vi "Monitor and Configure Time References.vi"() -> ()   [LabVIEW 2019]
doc: "Demonstrates how to monitor and configure IEEE 1588-2008 and IEEE 802.1AS-2011 time references running on a real-time system."
uses:
  <instrlib>/niSync/niSync.llb/niSync Initialize (Default).vi
panel:
  out "Timing:Offset from Time Reference (ns)":dbl
  in  "BMCA Mode":i32(ring) items=["SlaveOnly", "MasterSlave"]
  in  "NI-Sync Resource":tag
  out "Error Out":errorcluster
  in  "stop":bool
  in  "802.1AS:Clock Accuracy":i32(ring)=32 items=["Within25nsec"=32, "Within100nsec"=33, "Within250nsec"=34, "Within1usec"=35, "Within2500nsec"=36, "Within10usec"=37, "Within25usec"=38, "Within100usec"=39, "Within250usec"=40, "Within1msec"=41, "Within2500usec"=42, "Within10msec"=43, "Within25msec"=44, "Within100msec"=45, "Within250msec"=46, "Within1sec"=47, "Within10sec"=48, "GreaterThan10sec"=49, "Unknown"=254]
  in  "Port State":i32(ring)=3 items=["Disabled"=3, "Master"=6, "Passive"=7, "Slave"=9]
  in  "1588:Clock Accuracy":i32(ring) items=["Unknown", "Within25nsec", "Within100nsec", "Within250nsec", "Within1usec", "Within2500nsec", "Within10usec", "Within25usec", "Within100usec", "Within250usec", "Within1msec", "Within2500usec", "Within10msec", "Within25msec", "Within100msec", "Within250msec", "Within1sec", "Within10sec", "GreaterThan10sec"]
  in  "Clock State":i32(ring) items=["Initializing", "Faulty", "Disabled", "Listening", "PreMaster", "Master", "Passive", "Uncalibrated", "Slave", "Stopped"]
  in  "Protocol Tab":T1(tab) caption="System Properties"
  in  "Persist?":bool
  out "802.1AS Monitor":string[][](table)
  in  "802.1AS Time Reference to Configure":i32(ring)
  in  "Priority1":i32=246
  in  "Priority2":i32=247
  in  "Apply 802.1as":bool caption="stop"
  out "802.1AS TAB Monitor":string[][](table)
  in  "Apply 802.1as TAB":bool caption="stop"
  in  "Persist?":bool
  in  "Priority2":i32=247
  in  "Priority1":i32=246
  in  "802.1AS TAB Time Reference to Configure":i32(ring)
  in  "Persist?":bool
  in  "1588 Time Reference to Configure":i32(ring) items=["IEEE 1588-2008_2"]
  in  "Appy 1588":bool caption="stop"
  out "1588 Monitor":string[][](table)
  in  "Priority1":i32=128
  in  "Priority2":i32=128
  in  "BMCA Mode":i32(ring)=1 items=["SlaveOnly", "MasterSlave"]
  out "1588 BC Monitor":string[][](table)
  in  "Appy 1588 BC":bool caption="stop"
  in  "Persist?":bool
  in  "Priority2":i32=128
  in  "Priority1":i32=128
  in  "1588 BC Time Reference to Configure":i32(ring)
  # "Setup"
  # "Overview: Demonstrates how to monitor and configure IEEE 1588-2008 (BC) and IEEE 802.1AS-2011 (TAB)\ntime references running on a real-time system.\nRequirements: Runs on Windows and Linux RT hosts to configure and monitor Linux RT devices.\nInstructions:\n1. Select the resource to monitor/configure in the NI-Sync Resource dropdown.\n2. Select the desired polling interval for monitoring.\n3. Use the tabs to switch to the protcol of interest.\n4. Monitor the enabled time references of this type in the table.\n5. To configure properties of a time reference:\n     a) Select the 1588 Time Reference to Configure.\n     b) Set properties to desired values.\n     c) Enable the Persist? Boolean if you would like these settings to persist across reboots.\n     d) Select Apply to commit the desired settings."
  # "IEEE 802.1AS-2011 is a network-based time synchronization protocol that is similar to IEEE 1588-2008, but is optimized for time-sensitive applications. It also provides fewer configuration options and\nrequires 802.1AS-compatible network infrastructure. Each instance of IEEE 802.1AS-2011 is associated with a single network interface on the real-time system, and each can be either a slave to the\nnetwork's grandmaster or the grandmaster to a network of devices."
  # "IEEE 802.1AS-2011 TAB (time-aware bridge) is like IEEE 802.1AS-2011, except each instance of IEEE 802.1AS-2011 TAB is associated with multiple ports, typically on a device that acts as a network switch."
  # "IEEE 1588-2008 is a network-based time synchronization protocol (also refered to as PTP) that synchronized devices to a single grandmaster clock. Each instance of IEEE 1588-2008 is associated with a\nsingle network interface on the real-time system, and each can be either a slave to the network's grandmaster or the grandmaster to a network of devices."
  # "IEEE 1588-2008 BC (boundary clock) is like IEEE 1588-2008, except each instance of IEEE 1588-2008 BC is associated with multiple ports, typically on a device that acts as a network switch."
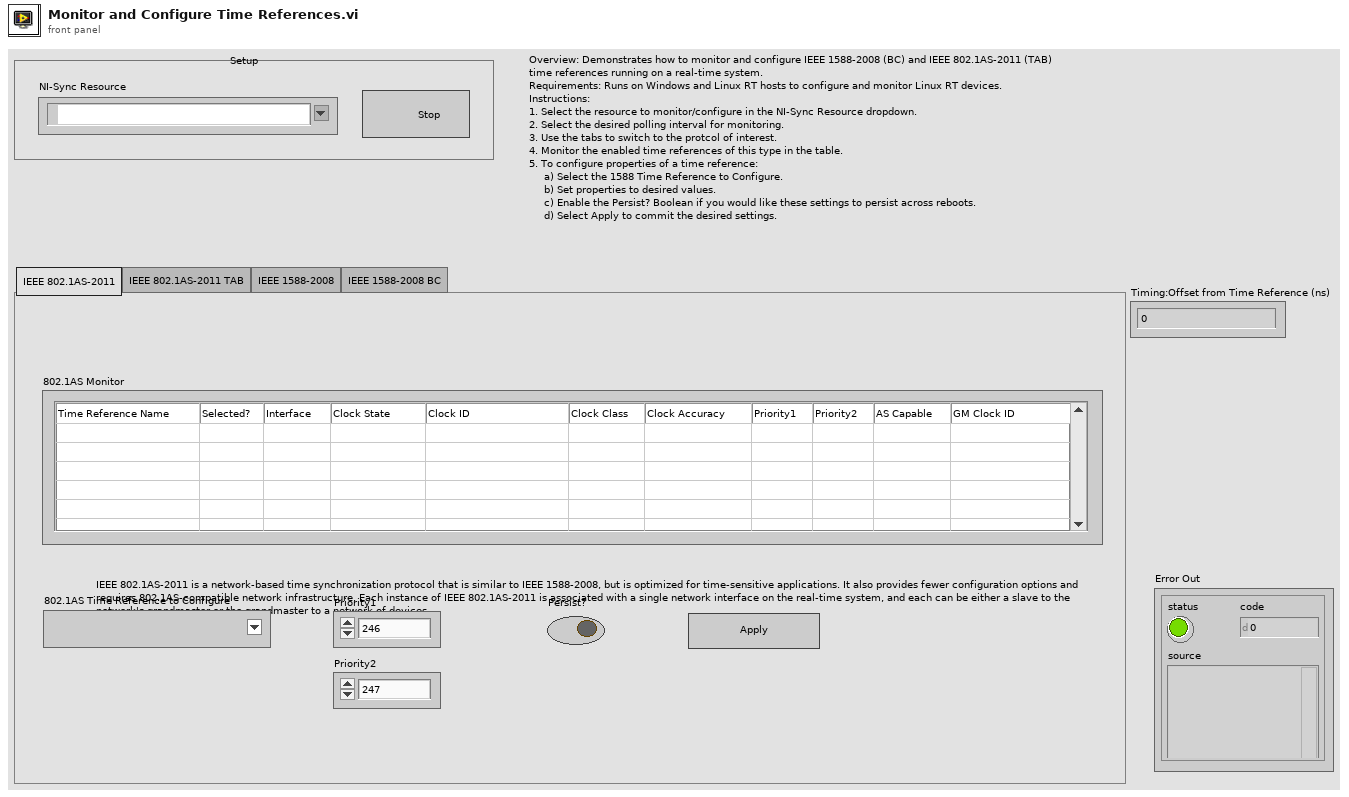
[diagram p1: front panel]
types:
  T1 = enum32{"IEEE 802.1AS-2011", "IEEE 802.1AS-2011 TAB", "IEEE 1588-2008", "IEEE 1588-2008 BC"}
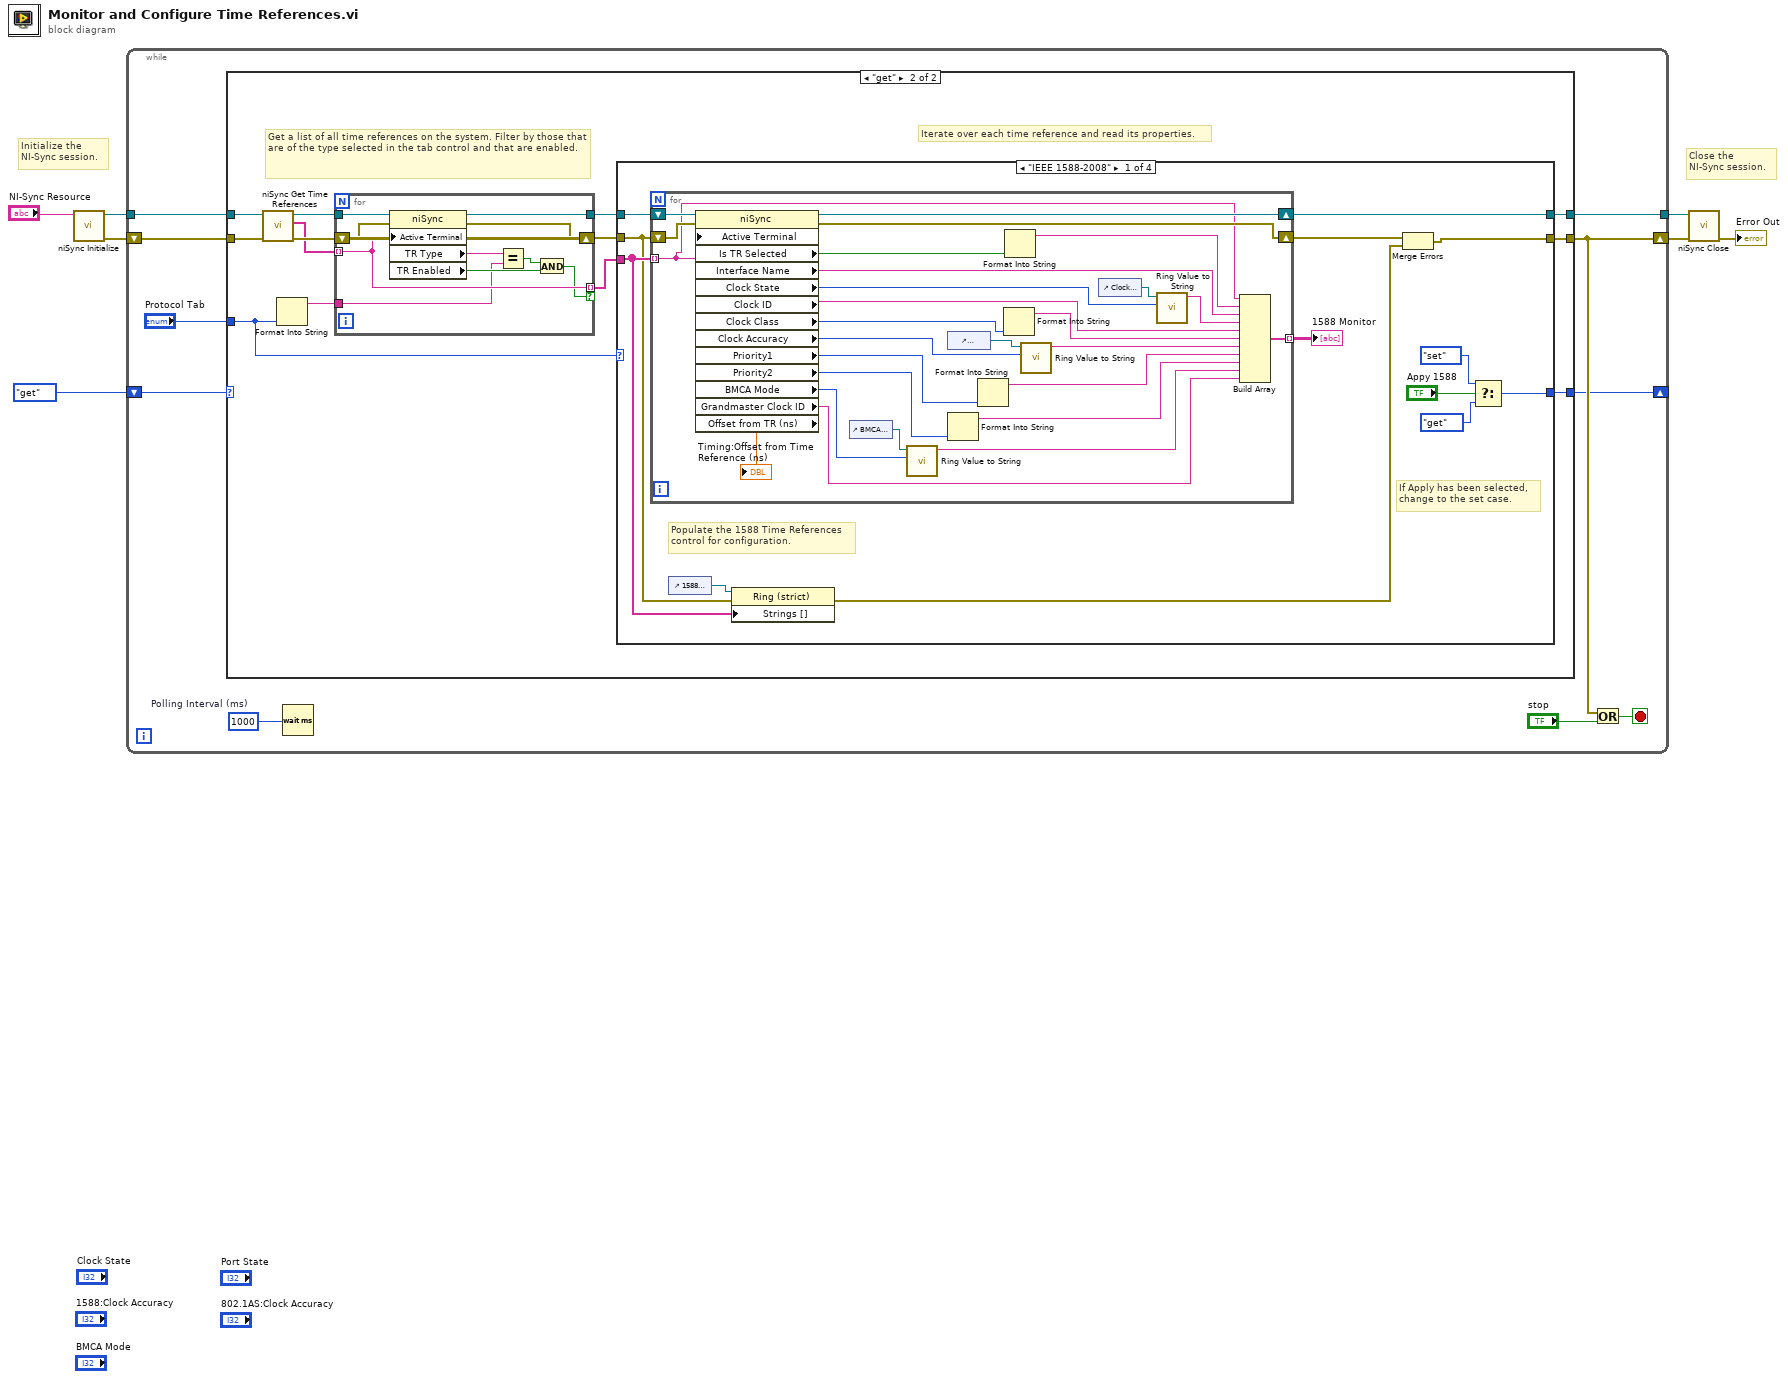
[diagram p0: block diagram]
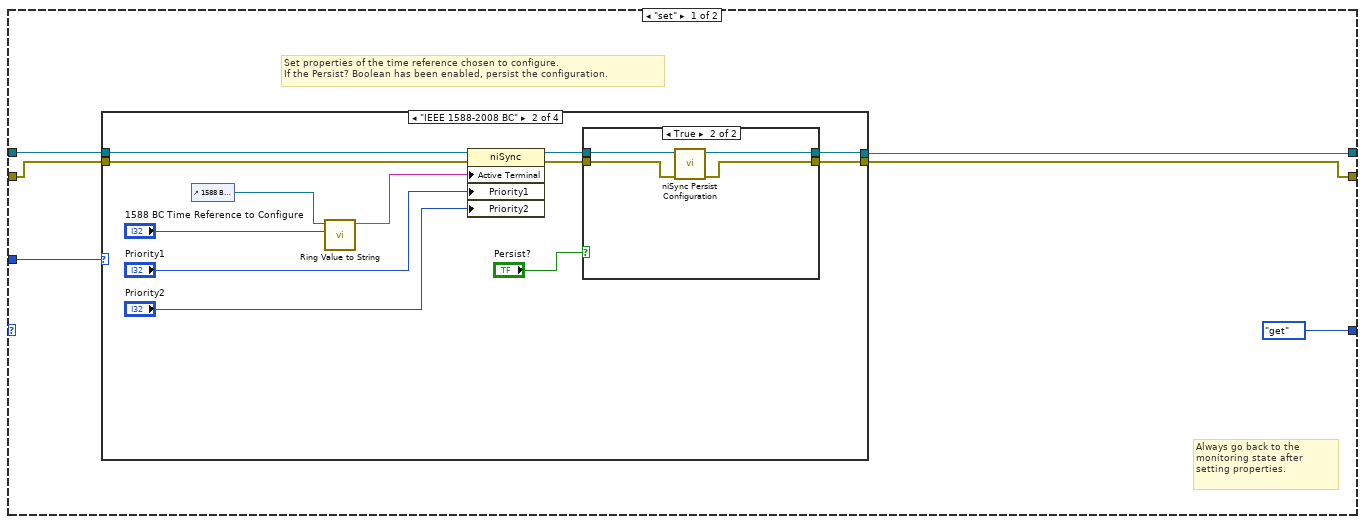
[diagram p2: hidden frame]
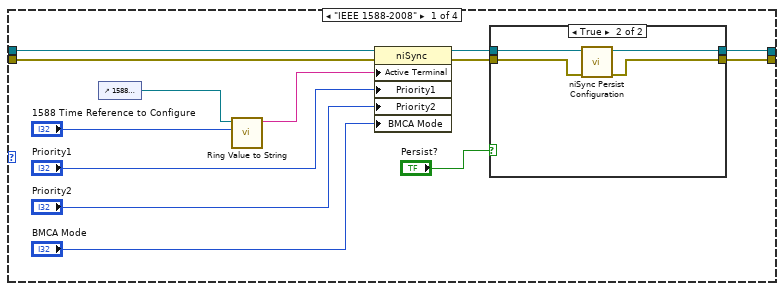
[diagram p3: hidden frame]
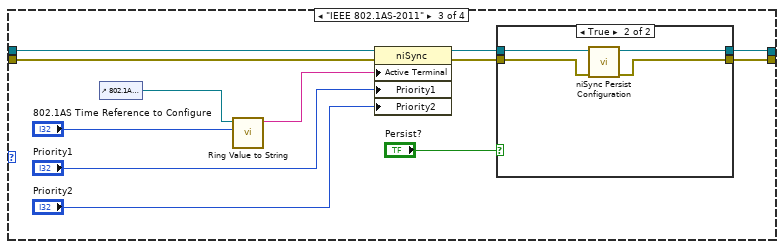
[diagram p6: hidden frame]
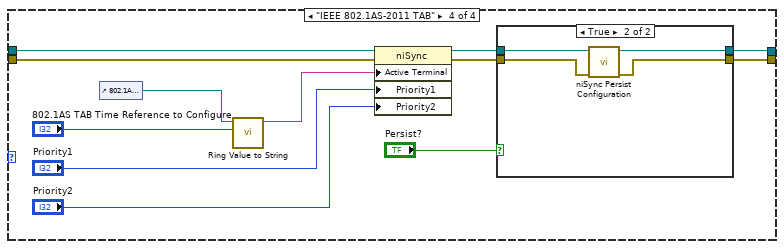
[diagram p8: hidden frame]
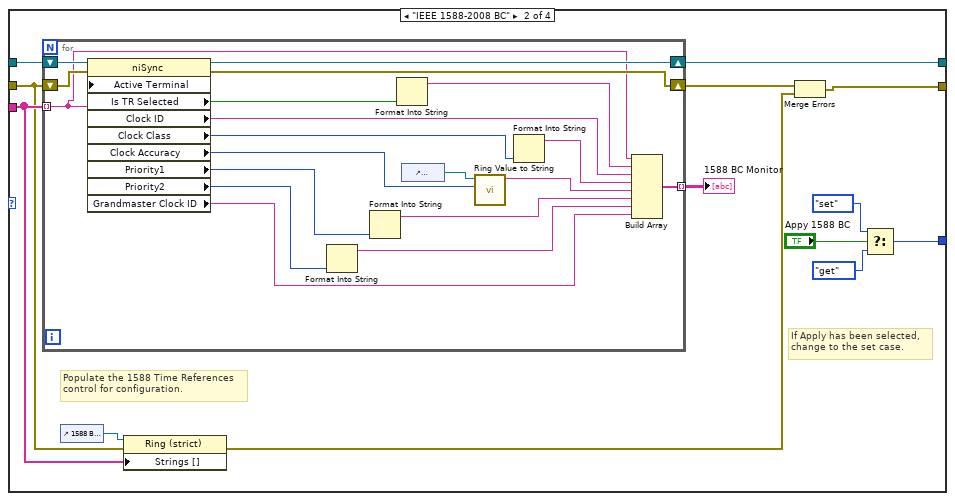
[diagram p10: hidden frame]
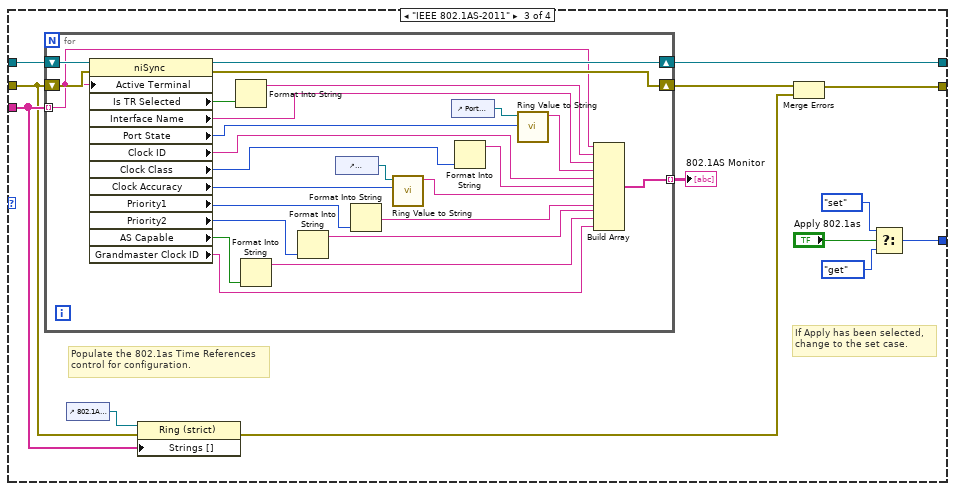
[diagram p11: hidden frame]
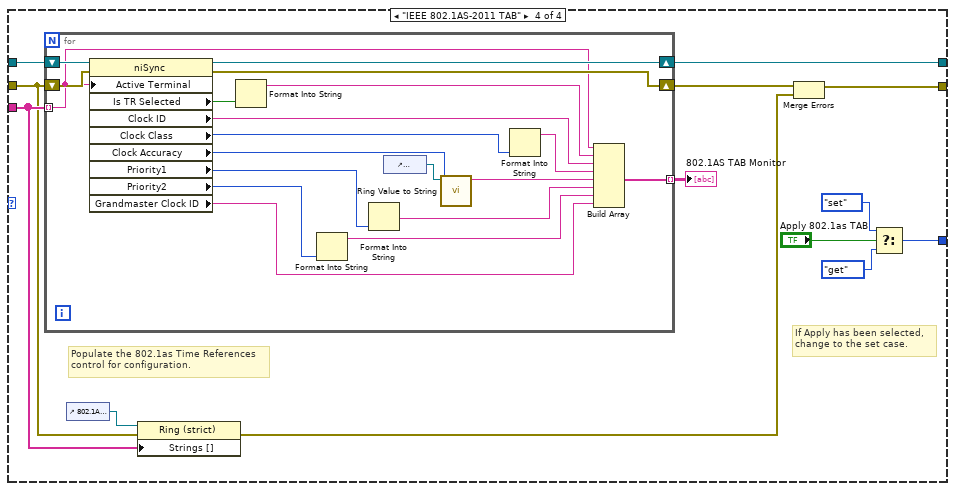
[diagram p12: hidden frame]
diagram:
  # "Close the\nNI-Sync session."
  # "Initialize the\nNI-Sync session."
  n1 = call-poly <instrlib>:"niSync Initialize.vi"("resource name"="NI-Sync Resource") -> ("error out"=w5:errorcluster, "instrument handle out"=w7:refnum<k15>)  [unwired: 9 in]
  n2 = while {
    tunnel: w7 -> [w17]
    tunnel: [w15] -> w6
    shift-right: [w13] -> w4
    shift-left: w5 -> [w16]
    shift-right: [w8] -> _
    shift-left: enum16{"get", "set"}."get" -> [w10]
    stop <- w14 stop-if-true
    w12 = u32 1000  # Polling Interval (ms)
    n3 = case shown="\"get\"" w10 {
      tunnel: w17 -> [w23 w109]
      tunnel: w16 -> [w19 w108]
      tunnel: [w22 w103] -> w15
      tunnel: [w21 w98] -> w13
      tunnel: "Protocol Tab" -> [w20 w99]
      tunnel: [enum16{"get", "set"}."get" w97] -> w8
      frame "set" {
        # "Always go back to the\nmonitoring state after setting properties."
        # "Set properties of the time reference chosen to configure.\nIf the Persist? Boolean has been enabled, persist the configuration."
        n4 = case shown="\"IEEE 1588-2008 BC\"" w20 {
          tunnel: w23 -> [w34 w52 w67 w85]
          tunnel: [w28 w46 w62 w80] -> w22
          tunnel: w19 -> [w30 w48 w66 w84]
          tunnel: [w27 w45 w61 w79] -> w21
          frame "IEEE 1588-2008" {
            n5 = control-ref of="1588 Time Reference to Configure"() -> (w36:refnum<vi>)
            n6 = call "Ring Value to String.vi"("Value"="1588 Time Reference to Configure", "Ring in"=w36) -> ("String"=w33:string)  [unwired: 9 in]
            n7 = property class="niSync"(reference=w34, error in=w30, "Active Terminal"=w33, "Priority1"="Priority1", "Priority2"="Priority2", "BMCA Mode"="BMCA Mode") -> (reference out=w29:refnum<k15>, error out=w26:errorcluster)
            n8 = case shown="True" "Persist?" {
              tunnel: [w38 w42] -> w28
              tunnel: [w37 w41] -> w27
              tunnel: w29 -> [w38 w40]
              tunnel: w26 -> [w37 w39]
              frame False {
              }
              frame True {
                n9 = call <instrlib>:"niSync Persist Configuration.vi"("error in (no error)"=w39, "instrument handle"=w40) -> ("error out"=w41:errorcluster, "instrument handle out"=w42:refnum<k15>)  [unwired: 8 in]
              }
            }
          }
          frame "IEEE 1588-2008 BC" {
            n10 = control-ref of="1588 BC Time Reference to Configure"() -> (w54:refnum<vi>)
            n11 = call "Ring Value to String.vi"("Value"="1588 BC Time Reference to Configure", "Ring in"=w54) -> ("String"=w51:string)  [unwired: 9 in]
            n12 = property class="niSync"(reference=w52, error in=w48, "Active Terminal"=w51, "Priority1"="Priority1", "Priority2"="Priority2") -> (reference out=w47:refnum<k15>, error out=w44:errorcluster)
            n13 = case shown="True" "Persist?" {
              tunnel: [w56 w60] -> w46
              tunnel: [w55 w59] -> w45
              tunnel: w47 -> [w56 w58]
              tunnel: w44 -> [w55 w57]
              frame False {
              }
              frame True {
                n14 = call <instrlib>:"niSync Persist Configuration.vi"("error in (no error)"=w57, "instrument handle"=w58) -> ("error out"=w59:errorcluster, "instrument handle out"=w60:refnum<k15>)  [unwired: 8 in]
              }
            }
          }
          frame "IEEE 802.1AS-2011" {
            n15 = control-ref of="802.1AS Time Reference to Configure"() -> (w72:refnum<vi>)
            n16 = call "Ring Value to String.vi"("Value"="802.1AS Time Reference to Configure", "Ring in"=w72) -> ("String"=w68:string)  [unwired: 9 in]
            n17 = property class="niSync"(reference=w67, error in=w66, "Active Terminal"=w68, "Priority1"="Priority1", "Priority2"="Priority2") -> (reference out=w64:refnum<k15>, error out=w63:errorcluster)
            n18 = case shown="True" "Persist?" {
              tunnel: w64 -> [w74 w78]
              tunnel: w63 -> [w73 w77]
              tunnel: [w74 w76] -> w62
              tunnel: [w73 w75] -> w61
              frame False {
              }
              frame True {
                n19 = call <instrlib>:"niSync Persist Configuration.vi"("error in (no error)"=w77, "instrument handle"=w78) -> ("error out"=w75:errorcluster, "instrument handle out"=w76:refnum<k15>)  [unwired: 8 in]
              }
            }
          }
          frame "IEEE 802.1AS-2011 TAB" {
            n20 = control-ref of="802.1AS TAB Time Reference to Configure"() -> (w90:refnum<vi>)
            n21 = call "Ring Value to String.vi"("Value"="802.1AS TAB Time Reference to Configure", "Ring in"=w90) -> ("String"=w86:string)  [unwired: 9 in]
            n22 = property class="niSync"(reference=w85, error in=w84, "Active Terminal"=w86, "Priority1"="Priority1", "Priority2"="Priority2") -> (reference out=w82:refnum<k15>, error out=w81:errorcluster)
            n23 = case shown="True" "Persist?" {
              tunnel: w82 -> [w92 w96]
              tunnel: w81 -> [w91 w95]
              tunnel: [w92 w94] -> w80
              tunnel: [w91 w93] -> w79
              frame False {
              }
              frame True {
                n24 = call <instrlib>:"niSync Persist Configuration.vi"("error in (no error)"=w95, "instrument handle"=w96) -> ("error out"=w93:errorcluster, "instrument handle out"=w94:refnum<k15>)  [unwired: 8 in]
              }
            }
          }
        }
      }
      frame "get" {
        # "Iterate over each time reference and read its properties."
        # "Get a list of all time references on the system. Filter by those that are of the type selected in the tab control and that are enabled."
        n25 = call <instrlib>:"niSync Get Time References.vi"("error in (no error)"=w108, "instrument handle"=w109) -> ("error out"=w106:errorcluster, "time references"=w105:string[], "instrument handle out"=w107:refnum<k15>)  [unwired: 7 in]
        n26 = Format Into String(w99) -> (resulting string=w100:string)  [unwired: 3 in, 1 out]
        n27 = for {
          tunnel: w107 -> [w261]
          tunnel: w105 -> [w258] mode=indexing
          tunnel: w100 -> [w252]
          tunnel: [w258] -> w104 mode=indexing if=w254
          tunnel: [w257] -> w102
          shift-right: [w253] -> w101
          shift-left: w106 -> [w260]
          n28 = property class="niSync"(reference=w261, error in=w260, "Active Terminal"=w258) -> (reference out=w257:refnum<k15>, error out=w253:errorcluster, "TR Type"=w259:string, "TR Enabled"=w255:bool)
          n29 = Equal?(x=w259, y=w252) -> (x = y?=w256:bool)
          n30 = And(x=w256, y=w255) -> (x .and. y?=w254:bool)
        }
        n31 = case shown="\"IEEE 1588-2008\"" w99 {
          tunnel: w104 -> [w118 w158 w191 w229]
          tunnel: w102 -> [w122 w162 w194 w232]
          tunnel: [w121 w161 w193 w231] -> w103
          tunnel: w101 -> [w115 w155 w186 w224]
          tunnel: [w114 w154 w189 w227] -> w98
          tunnel: [w110 w150 w183 w221] -> w97
          frame "IEEE 1588-2008" {
            # "If Apply has been selected,\nchange to the set case."
            # "Populate the 1588 Time References\ncontrol for configuration."
            n32 = for {
              tunnel: w118 -> [w125] mode=indexing
              shift-right: [w129] -> w117
              shift-left: w115 -> [w147]
              tunnel: [w146] -> w120 mode=indexing
              shift-right: [w148] -> w121
              shift-left: w122 -> [w149]
              n33 = property class="niSync"(reference=w149, error in=w147, "Active Terminal"=w125) -> (reference out=w148:refnum<k15>, error out=w129:errorcluster, "Is TR Selected"=w127:bool, "Interface Name"=w128:string, "Clock State"=w142:i32, "Clock ID"=w140:string, "Clock Class"=w145:i32, "Clock Accuracy"=w144:i32, "Priority1"=w143:i32, "Priority2"=w134:i32, "BMCA Mode"=w133:i32, "Grandmaster Clock ID"=w132:string, "Offset from TR (ns)"=→"Timing:Offset from Time Reference (ns)":dbl)
              n34 = control-ref of="BMCA Mode"() -> (w124:refnum<vi>)
              n35 = call "Ring Value to String.vi"("Value"=w133, "Ring in"=w124) -> ("String"=w131:string)  [unwired: 9 in]
              n36 = control-ref of="1588:Clock Accuracy"() -> (w135:refnum<vi>)
              n37 = Format Into String(w134) -> (resulting string=w136:string)  [unwired: 3 in, 1 out]
              n38 = Format Into String(w143) -> (resulting string=w137:string)  [unwired: 3 in, 1 out]
              n39 = Format Into String(w145) -> (resulting string=w139:string)  [unwired: 3 in, 1 out]
              n40 = Format Into String(w127) -> (resulting string=w126:string)  [unwired: 3 in, 1 out]
              n41 = call "Ring Value to String.vi"("Value"=w144, "Ring in"=w135) -> ("String"=w138:string)  [unwired: 9 in]
              n42 = control-ref of="Clock State"() -> (w130:refnum<vi>)
              n43 = call "Ring Value to String.vi"("Value"=w142, "Ring in"=w130) -> ("String"=w141:string)  [unwired: 9 in]
              n44 = Build Array(w125, w126, w128, w141, w140, w139, w138, w137, w136, w131, w132) -> (w146:string[])
            }
            "1588 Monitor" <- w120
            n45 = control-ref of="1588 Time Reference to Configure"() -> (w119:refnum<vi>)
            n46 = property on="Property Node" class="Ring (strict)"(reference=w119, error in=w115, "Strings []"=w118) -> (error out=w116:errorcluster)  [unwired: 1 out]
            n47 = Merge Errors(w117, w116) -> (w114:errorcluster)
            n48 = Select(t=enum16{"get", "set"}."set", s="Appy 1588", f=enum16{"get", "set"}."get") -> (s? t:f=w110:enum16{"get", "set"})
          }
          frame "IEEE 1588-2008 BC" {
            # "If Apply has been selected,\nchange to the set case."
            # "Populate the 1588 Time References\ncontrol for configuration."
            n49 = for {
              tunnel: w158 -> [w164] mode=indexing
              shift-right: [w167] -> w157
              shift-left: w155 -> [w179]
              tunnel: [w178] -> w160 mode=indexing
              shift-right: [w180] -> w161
              shift-left: w162 -> [w181]
              n50 = property class="niSync"(reference=w181, error in=w179, "Active Terminal"=w164) -> (reference out=w180:refnum<k15>, error out=w167:errorcluster, "Is TR Selected"=w166:bool, "Clock ID"=w163:string, "Clock Class"=w177:i32, "Clock Accuracy"=w176:i32, "Priority1"=w175:i32, "Priority2"=w169:i32, "Grandmaster Clock ID"=w168:string)
              n51 = Format Into String(w169) -> (resulting string=w171:string)  [unwired: 3 in, 1 out]
              n52 = Format Into String(w175) -> (resulting string=w172:string)  [unwired: 3 in, 1 out]
              n53 = Format Into String(w166) -> (resulting string=w165:string)  [unwired: 3 in, 1 out]
              n54 = control-ref of="1588:Clock Accuracy"() -> (w170:refnum<vi>)
              n55 = call "Ring Value to String.vi"("Value"=w176, "Ring in"=w170) -> ("String"=w173:string)  [unwired: 9 in]
              n56 = Format Into String(w177) -> (resulting string=w174:string)  [unwired: 3 in, 1 out]
              n57 = Build Array(w164, w165, w163, w174, w173, w172, w171, w168) -> (w178:string[])
            }
            "1588 BC Monitor" <- w160
            n58 = control-ref of="1588 BC Time Reference to Configure"() -> (w159:refnum<vi>)
            n59 = property on="Property Node" class="Ring (strict)"(reference=w159, error in=w155, "Strings []"=w158) -> (error out=w156:errorcluster)  [unwired: 1 out]
            n60 = Merge Errors(w157, w156) -> (w154:errorcluster)
            n61 = Select(t=enum16{"get", "set"}."set", s="Appy 1588 BC", f=enum16{"get", "set"}."get") -> (s? t:f=w150:enum16{"get", "set"})
          }
          frame "IEEE 802.1AS-2011" {
            # "If Apply has been selected,\nchange to the set case."
            # "Populate the 802.1as Time References\ncontrol for configuration."
            n62 = for {
              shift-right: [w205] -> w190
              shift-left: w186 -> [w218]
              tunnel: w191 -> [w203] mode=indexing
              tunnel: [w216] -> w192 mode=indexing
              shift-right: [w217] -> w193
              shift-left: w194 -> [w219]
              n63 = property class="niSync"(reference=w219, error in=w218, "Active Terminal"=w203) -> (reference out=w217:refnum<k15>, error out=w205:errorcluster, "Is TR Selected"=w202:bool, "Interface Name"=w204:string, "Port State"=w215:i32, "Clock ID"=w197:string, "Clock Class"=w195:i32, "Clock Accuracy"=w198:i32, "Priority1"=w211:i32, "Priority2"=w210:i32, "AS Capable"=w208:bool, "Grandmaster Clock ID"=w200:string)
              n64 = Format Into String(w202) -> (resulting string=w201:string)  [unwired: 3 in, 1 out]
              n65 = Format Into String(w208) -> (resulting string=w207:string)  [unwired: 3 in, 1 out]
              n66 = Format Into String(w210) -> (resulting string=w209:string)  [unwired: 3 in, 1 out]
              n67 = control-ref of="802.1AS:Clock Accuracy"() -> (w206:refnum<vi>)
              n68 = Format Into String(w211) -> (resulting string=w199:string)  [unwired: 3 in, 1 out]
              n69 = call "Ring Value to String.vi"("Value"=w198, "Ring in"=w206) -> ("String"=w212:string)  [unwired: 9 in]
              n70 = control-ref of="Port State"() -> (w196:refnum<vi>)
              n71 = Format Into String(w195) -> (resulting string=w213:string)  [unwired: 3 in, 1 out]
              n72 = call "Ring Value to String.vi"("Value"=w215, "Ring in"=w196) -> ("String"=w214:string)  [unwired: 9 in]
              n73 = Build Array(w203, w201, w204, w214, w197, w213, w212, w199, w209, w207, w200) -> (w216:string[])
            }
            "802.1AS Monitor" <- w192
            n74 = control-ref of="802.1AS Time Reference to Configure"() -> (w187:refnum<vi>)
            n75 = property on="Property Node" class="Ring (strict)"(reference=w187, error in=w186, "Strings []"=w191) -> (error out=w188:errorcluster)  [unwired: 1 out]
            n76 = Merge Errors(w190, w188) -> (w189:errorcluster)
            n77 = Select(t=enum16{"get", "set"}."set", s="Apply 802.1as", f=enum16{"get", "set"}."get") -> (s? t:f=w183:enum16{"get", "set"})
          }
          frame "IEEE 802.1AS-2011 TAB" {
            # "If Apply has been selected,\nchange to the set case."
            # "Populate the 802.1as Time References\ncontrol for configuration."
            n78 = for {
              shift-right: [w241] -> w228
              shift-left: w224 -> [w250]
              tunnel: w229 -> [w240] mode=indexing
              tunnel: [w248] -> w230 mode=indexing
              shift-right: [w249] -> w231
              shift-left: w232 -> [w251]
              n79 = property class="niSync"(reference=w251, error in=w250, "Active Terminal"=w240) -> (reference out=w249:refnum<k15>, error out=w241:errorcluster, "Is TR Selected"=w239:bool, "Clock ID"=w235:string, "Clock Class"=w234:i32, "Clock Accuracy"=w236:i32, "Priority1"=w245:i32, "Priority2"=w244:i32, "Grandmaster Clock ID"=w237:string)
              n80 = Format Into String(w239) -> (resulting string=w238:string)  [unwired: 3 in, 1 out]
              n81 = Format Into String(w244) -> (resulting string=w243:string)  [unwired: 3 in, 1 out]
              n82 = Format Into String(w245) -> (resulting string=w233:string)  [unwired: 3 in, 1 out]
              n83 = control-ref of="802.1AS:Clock Accuracy"() -> (w242:refnum<vi>)
              n84 = call "Ring Value to String.vi"("Value"=w236, "Ring in"=w242) -> ("String"=w246:string)  [unwired: 9 in]
              n85 = Format Into String(w234) -> (resulting string=w247:string)  [unwired: 3 in, 1 out]
              n86 = Build Array(w240, w238, w235, w247, w246, w233, w243, w237) -> (w248:string[])
            }
            "802.1AS TAB Monitor" <- w230
            n87 = control-ref of="802.1AS TAB Time Reference to Configure"() -> (w225:refnum<vi>)
            n88 = property on="Property Node" class="Ring (strict)"(reference=w225, error in=w224, "Strings []"=w229) -> (error out=w226:errorcluster)  [unwired: 1 out]
            n89 = Merge Errors(w228, w226) -> (w227:errorcluster)
            n90 = Select(t=enum16{"get", "set"}."set", s="Apply 802.1as TAB", f=enum16{"get", "set"}."get") -> (s? t:f=w221:enum16{"get", "set"})
          }
        }
      }
    }
    n91 = Wait (ms)(milliseconds to wait=w12) -> ()  [unwired: 1 out]
    n92 = Or(x=w13, y="stop") -> (x .or. y?=w14:bool)
  }
  n93 = call <instrlib>:"niSync Close.vi"("error in (no error)"=w4, "instrument handle"=w6) -> ("error out"=→"Error Out":errorcluster)  [unwired: 9 in]
